vi "Update.vi"(0 "reference in":refnum<class "Save.lvclass">, 5 "error in (no error)":errorcluster) -> (14 "reference out":refnum<class "Save.lvclass">, 19 "error out":errorcluster)   [LabVIEW 2013, in "Save.lvclass"]
uses:
  Save.lvclass
  DAQ_class/DAQ.lvclass
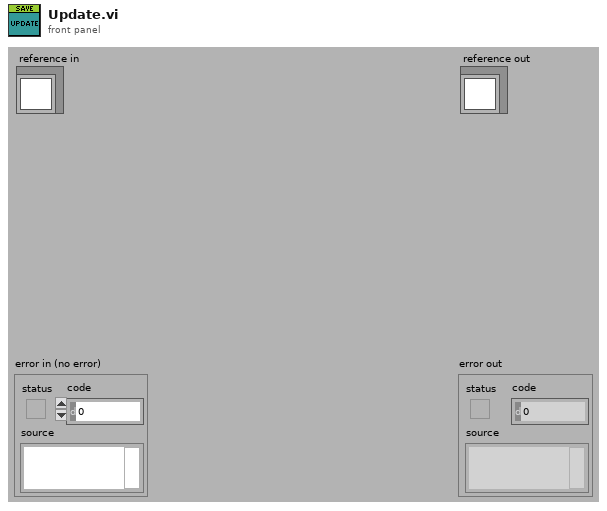
[diagram p1: front panel]
types:
  T1 = typedef "Save.lvclass/ObjectAttributes.ctl" = cluster{"DAQ.lvclass":refnum<class "DAQ.lvclass">}
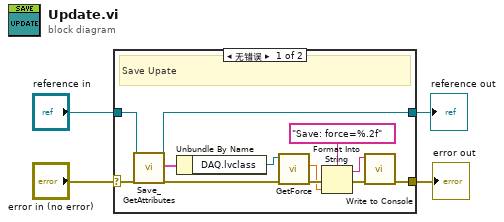
[diagram p0: block diagram]
diagram:
  n1 = case shown="无错误" "error in (no error)" {
    selector: "error in (no error)" -> [w16 w18]
    tunnel: [w6 w18] -> w3
    tunnel: [w15 w17] -> w1
    tunnel: "reference in" -> [w13 w17]
    frame No Error {
      # "Save Upate"
      n2 = call "Save_GetAttributes.vi"("reference in"=w13, "error in (no error)"=w16) -> ("reference out"=w15:refnum<class "Save.lvclass">, "attributes"=w14:T1, "error out"=w11:errorcluster)  [unwired: 14 in, 1 out]
      n3 = Unbundle By Name(w14) -> ("DAQ.lvclass"=w12:refnum<class "DAQ.lvclass">)
      n4 = call-dynamic "GetForce.vi"("error in (no error)"=w11, "reference in"=w12) -> ("error out"=w10:errorcluster, "Force"=w5:dbl)  [unwired: 7 in, 1 out]
      n5 = Format Into String(format string="Save: force=%.2f" ("格式字符串"), error in=w10, w5) -> (resulting string=w8:string, error out=w7:errorcluster)  [unwired: 1 in]
      n6 = call "Write to Console.vi"("error in (no error)"=w7, "Input"=w8) -> ("error out"=w6:errorcluster)  [unwired: 9 in]
    }
    frame Error {
    }
  }
  "error out" <- w3
  "reference out" <- w1
